vi "Create Container.vi"(8 "Error In":errorcluster, 11 "MDI Area Builder in":refnum<class "MDI Area Builder.lvclass">) -> (0 "Error Out":errorcluster, 2 "Container":refnum<class "QWidget.lvclass">, 3 "MDI Area Builder out":refnum<class "MDI Area Builder.lvclass">)   [LabVIEW 2014, in "MDI Area Builder.lvclass"]
doc: "Implements the interface provided by Abstract Widget Builder.\n\n\nCopyright (c) 2019 Sze Howe Koh.\nThis code is licensed under the MIT license."
uses:
  MDI Area Builder.lvclass
  <vilib>/addons/LQ/Qt Widgets/QWidget/QWidget.lvclass
  <vilib>/addons/LQ/LQ Core/Qt/ScrollBarPolicy.ctl
  <vilib>/addons/LQ/Qt Widgets/QAbstractScrollArea/setHorizontalScrollBarPolicy.vi
  <vilib>/addons/LQ/Qt Widgets/QAbstractScrollArea/setVerticalScrollBarPolicy.vi
  <vilib>/addons/LQ/Qt Widgets/QMdiArea/QMdiArea.lvclass
  <vilib>/addons/LQ/LQ Core/Qt/Qt.lvlib
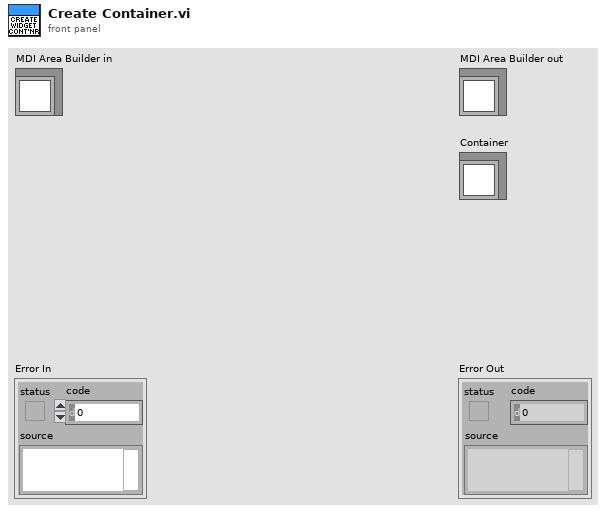
[diagram p1: front panel]
types:
  T1 = typedef "Qt.lvlib/ScrollBarPolicy.ctl" = i32
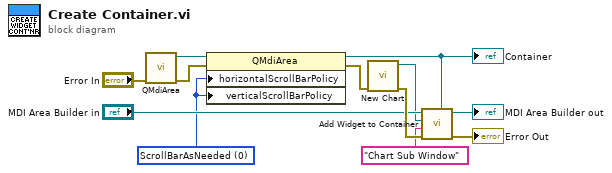
[diagram p0: block diagram]
diagram:
  w5 = T1 0 items=["ScrollBarAsNeeded", "ScrollBarAlwaysOff", "ScrollBarAlwaysOn"] ("horizontalScrollBarPolicy")
  n1 = call <vilib>:"QMdiArea.vi"("Error In"="Error In") -> ("Error Out"=w2:errorcluster, "New QMdiArea"=w4:refnum<class "QMdiArea.lvclass">)  [unwired: 9 in]
  n2 = property class="QMdiArea"(reference=w4, error in=w2, "horizontalScrollBarPolicy"=w5, "verticalScrollBarPolicy"=w5) -> (reference out=w3:refnum<class "QMdiArea.lvclass">, error out=w1:errorcluster)
  "Container" <- w3
  n3 = call "New Chart.vi"("Error In"=w1) -> ("Error Out"=w12:errorcluster, "New LQChart"=w7:refnum<class "LQChart.lvclass">)  [unwired: 9 in]
  n4 = call-dynamic "Add Widget to Container.vi"("Container"=w3, "Error In"=w12, "Label"="Chart Sub Window" ("windowTitle"), "Widget"=w7, "MDI Area Builder in"="MDI Area Builder in") -> ("Error Out"=→"Error Out":errorcluster, "MDI Area Builder out"=→"MDI Area Builder out":refnum<class "MDI Area Builder.lvclass">)  [unwired: 5 in]
